vi "Simple Read.vi"(4 "Abs_String in":refnum<class "Abs_String 1D.lvclass">) -> (1 "Array":string[](array[string]))   [LabVIEW 2021, in "Abs_String 1D.lvclass"]
uses:
  Abs_String 1D.lvclass
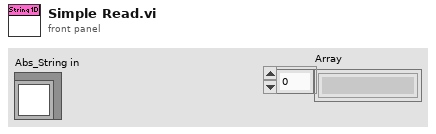
[diagram p1: front panel]
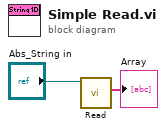
[diagram p0: block diagram]
diagram:
  n1 = call-dynamic "Read.vi"("Abs_String in"="Abs_String in") -> ("Array"=→"Array":string[])  [unwired: 8 in, 2 out]
